vi "Carbide-Global.vi"() -> ()   [LabVIEW 2014]
uses:
  <vilib>/httpClient/ClientHandle.ctl
  <vilib>/httpClient/LabVIEWHTTPClient.lvlib
panel:
  out "Refnum out":T1
  in  "Laser IP address":string
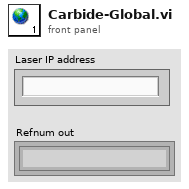
[diagram p1: front panel]
types:
  T1 = typedef "LabVIEWHTTPClient.lvlib/ClientHandle.ctl" = refnum<k1>
diagram:
